vi "Find Red Pitaya Digitizers VISA.vi"(6 "Timeout":i32=100, 7 "Logic tags":u16[](array[numeric])=[101, 102], 8 "Error In":errorcluster, 9 "End address":i32=120, 10 "Start address":i32=100, 11 "Subnet":string="192.168.1") -> (0 "Error Out":errorcluster, 1 "connections":refnum<visa-resource-name>[](array[refnum]), 2 "Device names":string[](array[string]), 3 "Digitizers out":refnum<class "Pulse Driver.lvclass">[](array[class]))   [LabVIEW 2016]
uses:
  Instruments/Pulse Driver/Pulse Driver.lvclass
  Red Pitaya Digitizer.lvclass
  C:/github/NHMFL_Core/Libraries/Instruments/Pulse Driver/Pulse Driver.lvclass
  Red Pitaya Digitizer.lvclass/Red Pitaya Digitizer.ctl
  RP Core/RP Instrument/RP Instrument.lvclass/RP Instrument.ctl
  Write Logic tag.vi
  Read RP Instrument.vi
  RP Core/RP Instrument/Write Samples per trigger increment .vi
  Write RP Instrument.vi
  Write Server address.vi
  RP Core/RP Instrument/RP Instrument.lvclass
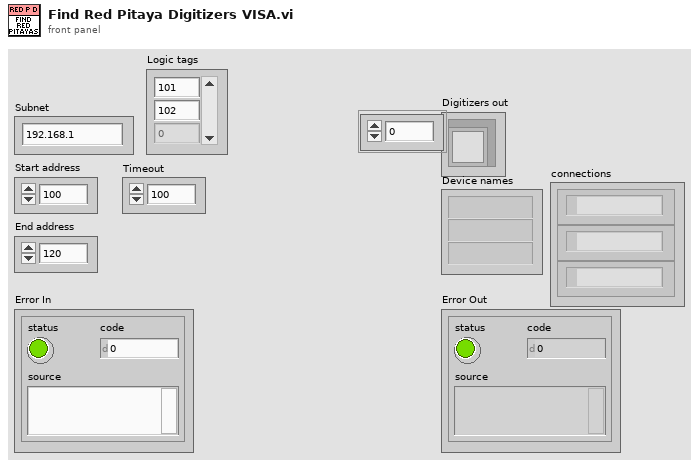
[diagram p1: front panel]
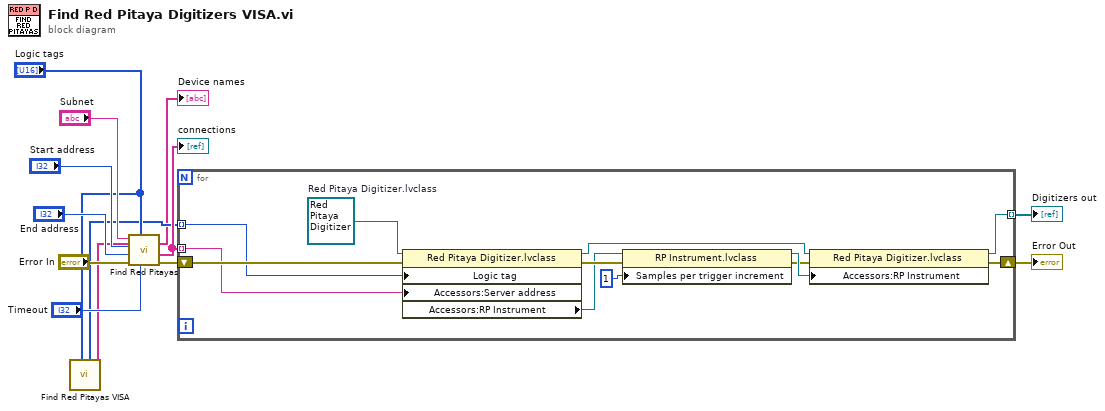
[diagram p0: block diagram]
diagram:
  n1 = call "Find Red Pitayas VISA.vi"("Logic tags"="Logic tags") -> ("Device names"=→"Device names":string[], "Logic tags out"=w2:u16[])  [unwired: 7 in, 2 out]
  n2 = call "Find Red Pitayas.vi"("Timeout"="Timeout", "Logic tags"="Logic tags", "Error In"="Error In", "End address"="End address", "Start address"="Start address", "Subnet"="Subnet") -> ("Error Out"=w4:errorcluster, "Addresses"=w6:string[])  [unwired: 2 in, 2 out]
  "connections" <- w6
  n3 = for {
    tunnel: w6 -> [w14] mode=indexing
    shift-right: [w19] -> w12
    shift-left: w4 -> [w23]
    tunnel: [w15] -> w11 mode=indexing
    tunnel: w2 -> [w13] mode=indexing
    w24 = refnum<class "Red Pitaya Digitizer.lvclass"> refnum  # Red Pitaya Digitizer.lvclass
    n4 = property class="Red Pitaya Digitizer.lvclass"(reference=w24, error in=w23, "Logic tag"=w13, "Accessors:Server address"=w14) -> (reference out=w16:refnum<class "Red Pitaya Digitizer.lvclass">, error out=w22:errorcluster, "Accessors:RP Instrument"=w21:refnum<class "RP Instrument.lvclass">)
    n5 = property class="RP Instrument.lvclass"(reference=w21, error in=w22, "Samples per trigger increment "=1 ("Samples per trigger increment")) -> (reference out=w18:refnum<class "RP Instrument.lvclass">, error out=w17:errorcluster)
    n6 = property class="Red Pitaya Digitizer.lvclass"(reference=w16, error in=w17, "Accessors:RP Instrument"=w18) -> (reference out=w15:refnum<class "Red Pitaya Digitizer.lvclass">, error out=w19:errorcluster)
  }
  "Digitizers out" <- w11
  "Error Out" <- w12
